vi "1003088 print label from powered unit.vi"(8 "error in (no error)":errorcluster, 10 "Baud":dbl=115200.0, 11 "VISA Refnum in":refnum<visa-resource-name>="COM11") -> (0 "error out":errorcluster)   [LabVIEW 2013]
panel:
  in  "Check label IMEI to unit?":bool
  out "IP":string
  out "Print Label OK?":bool=TRUE
  in  "Serial Number":u32
  in  "Printer name":string="\\\\SkywireTestPC1\\ZDesigner ZT230-300dpi ZPL (Copy 1)"
  out "ZPL final":string
  in  "ZPL template":string="\u0010CT~~CD,~CC^~CT~\n^XA~TA000~JSN^LT0^MNW^MTT^PON^PMN^LH0,0^JMA^PR4,4~SD21^JUS^LRN^CI0^XZ\n^FX Start of label zpl^FS\n^XA\n^MMT\n^PW300\n^LL0300\n^LS0\n^FO30,20^GFA,01536,01536,00024,:Z64:\neJzt0s1Kw0AQAOC0gU3B0iB4EAlppQcvHlKE0kNhX0Uo6EsImVLwB8W+QLBvYtUFexH6AoJKhVwjuaSwdN100tDALiL04ME57OFjdnZ3Zg1jU2FB5Krc/kioyutxQkHpXO1zjXONL85+8AouZuaiS8Ere0s3oSsf5KAH0sm676G/UOgQI/OK9J3cD3NPG7OL/kmhTbYDtxJZA3BOJxd47ltE4YC0xv4WrzNwRDjE/KnsT5O0GKtVvV7qIyP3/fNWv39DjpvgfIX36BPZB+8Z/QicKEzQ2YJC40T6Zbngj2Llph+nztEfUm9jvlnwMXgu1l/6HfqTL6BRk35LvKYIonCYnUszv3Y6PfFadCL9KrGZCN5nVuYjsZpXaX1ebJp7YY4s1PhM47HG5xrnOvd/4/aAK/+/ZfKqyg2TK1nvQiQaV+6QvtiElzT1Dc19/uMPxjcSRcXX:E7E0\n\n^FO190,20^GFA,00256,00256,00008,:Z64:\neJxjYCAZMEFp/g8Q2v4PhK7gg9AJ7BD6/OMGEMV4/iOE7iuE0gUHwHT/Ayh9AEL3QfkwdecswTTDAeYGFHNh9sj/QXUHWQAAi6QYnQ==:D803\n\n^FT75,92^A0N,29,29^FH\\^FDSKYWIRE^FS\n^FO175,60^GFA,00256,00256,00008,:Z64:\neJxjYCAZMEFp/g8Q2v4PhK7gg9AJ7BD6/OMGEMV4/iOE7iuE0gUHwHT/Ayh9AEL3QfkwdecswTTDAeYGFHNh9sj/QXUHWQAAi6QYnQ==:D803\n\n^FT0,115^A@N,20,20,ari001^FH\\^FDP/N: NL-SW-LTE-TC1WWG^FS\n^FT0,139^A@N,23,23,ari001^FH\\^FDIMEI: ImeiImeiImeiIme^FS\n^FT0,163^A@N,19,19,ari001^FH\\^FDICCID:EsimEsimEsimEsimEsim^FS\n^FT0,187^A@N,19,19,ari001^FH\\^FDBTW BTWSNWWYY^FS\n^FT0,211^A@N,24,24,ari001^FH\\^FD1003088 REV A^FS\n^BY56,56^FT203,275^BXN,3,200,0,0,1,~\n^FH\\^FDImeiImeiImeiIme,BTW BTWSNWWYY,EsimEsimEsimEsimEsim^FS\n^PQ1,0,1,Y^XZ"
  out "imei":string
  out "eSim ICCID":string
  # "printer1=\\\\\\\\SkywireTestPC1\\ZDesigner ZT230-300dpi ZPL (Copy 1)\nprinter2=\\\\\\\\PucTestPC2\\ZDesigner ZT230-300dpi ZPL\nprinter3=\\\\\\\\NIMBELNKTESTPC3\\ZDesigner GX430t\nprinter4=\\\\\\\\dt-hkn77p2\\ZDesigner ZT230-200dpi ZPL\nprinter5=\\\\\\\\nimbelink-08\\ZDesigner ZT230-300dpi ZPL\nprinter6=\\\\\\\\LT-85LKFW2\\\\"
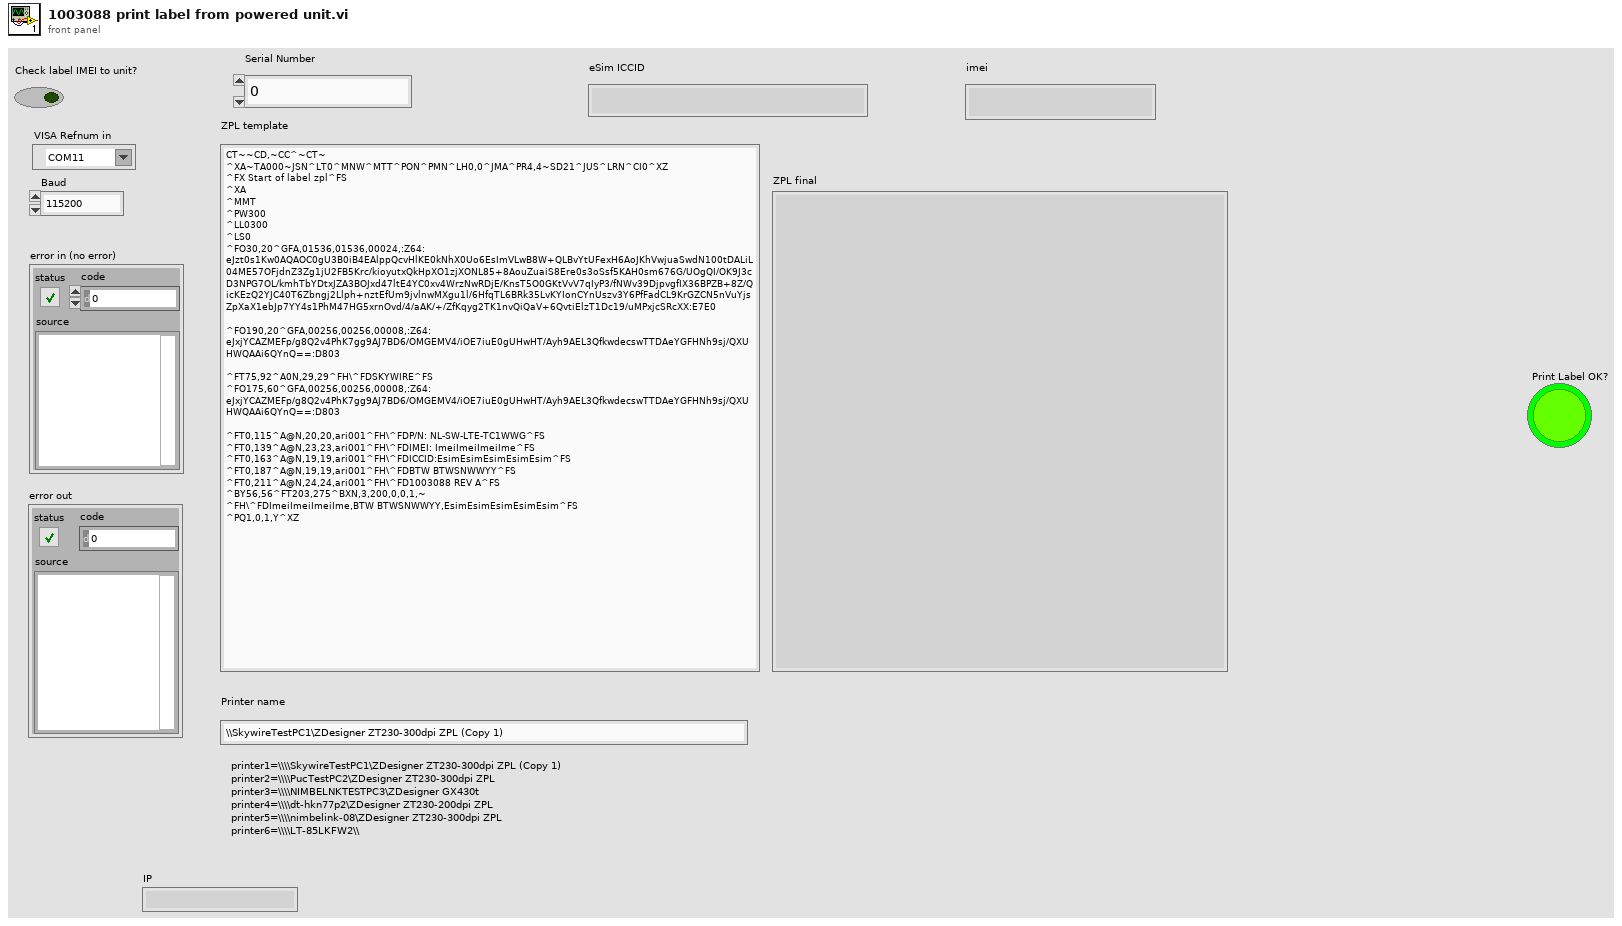
[diagram p1: front panel]
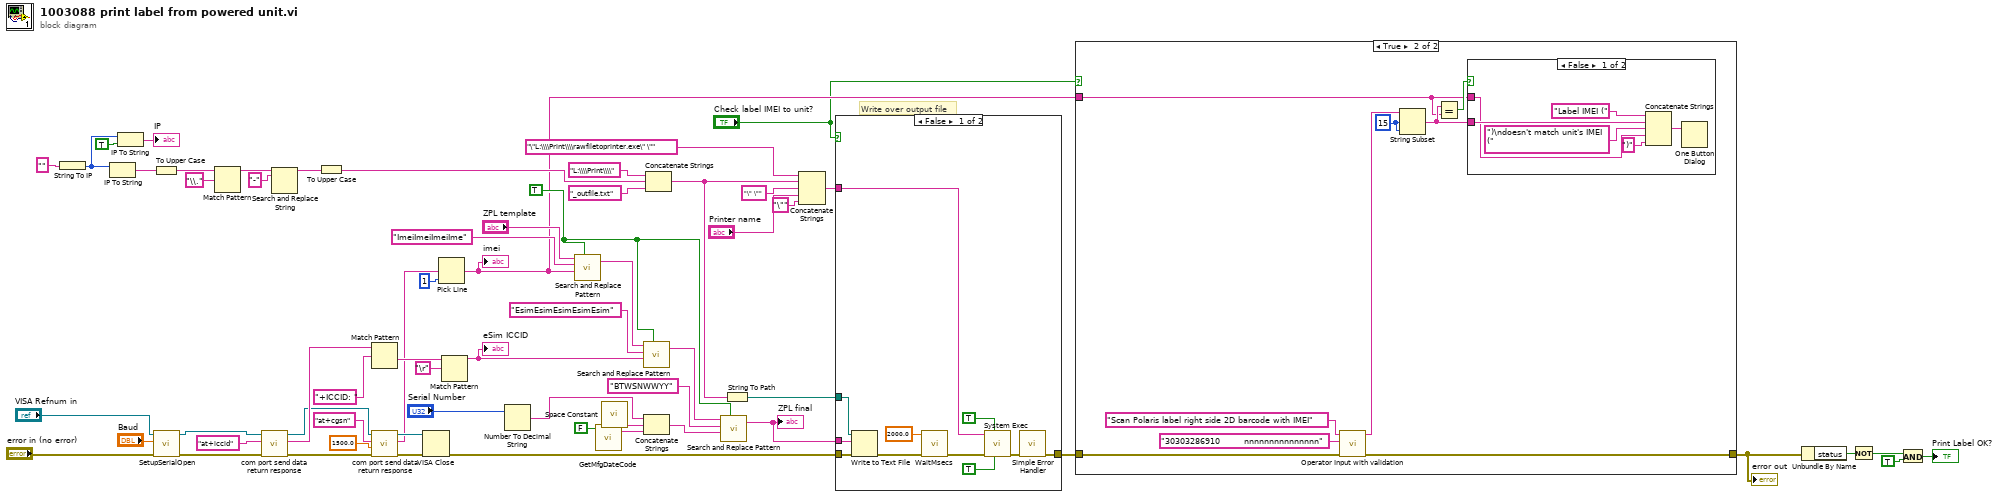
[diagram p0: block diagram]
diagram:
  w44 = TRUE ("replace all? (F)")
  # "Write over output file"
  n1 = String To IP(1:"" ("name")) -> (0:w28:u32)
  n2 = IP To String(2:w28) -> (0:w22:string)  [unwired: 1 in]
  n3 = IP To String(1:TRUE ("dot notation? (F)"), 2:w28) -> (0:→"IP":string)
  n4 = To Upper Case(1:w22) -> (0:w21:string)
  n5 = call "SetupSerialOpen.vi"("error in (no error)"="error in (no error)", "Baud"="Baud", "VISA Refnum in"="VISA Refnum in") -> ("error out"=w59:errorcluster, "VISA session"=w10:refnum<visa-resource-name>)  [unwired: 7 in]
  n6 = Match Pattern(string=w21, regular expression="\\.") -> (before substring=w25:string)  [unwired: 1 in, 3 out]
  n7 = call "com port send data return response.vi"("error in (no error)"=w59, "Send data"="at+iccid", "VISA resource name"=w10) -> ("error out"=w53:errorcluster, "response"=w55:string, "VISA resource name out"=w52:refnum<visa-resource-name>)  [unwired: 5 in, 1 out]
  n8 = Search and Replace String(input string=w25, search string="-") -> (result string=w23:string)  [unwired: 6 in, 3 out]
  n9 = To Upper Case(1:w23) -> (0:w20:string)
  n10 = Match Pattern(string=w55, regular expression="+ICCID: ") -> (after substring=w46:string)  [unwired: 1 in, 3 out]
  n11 = call "com port send data return response.vi"("error in (no error)"=w53, "Wait Msecs for response"=1500.0, "Send data"="at+cgsn", "VISA resource name"=w52) -> ("error out"=w41:errorcluster, "response"=w14:string, "VISA resource name out"=w51:refnum<visa-resource-name>)  [unwired: 4 in, 1 out]
  n12 = VISA Close(VISA resource name=w51, error in (no error)=w41) -> (error out=w17:errorcluster)
  n13 = Pick Line(multi-line string=w14, line index=1) -> (output string=w9:string)  [unwired: 1 in]
  "imei" <- w9
  n14 = Match Pattern(string=w46, regular expression="\r") -> (before substring=w11:string)  [unwired: 1 in, 3 out]
  "eSim ICCID" <- w11
  n15 = Number To Decimal String(number="Serial Number") -> (decimal integer string=w5:string)  [unwired: 1 in]
  n16 = call <vilib>:"Search and Replace Pattern.vi"("string"="ZPL template", "regular expression (\"\")"="ImeiImeiImeiIme" ("string"), "replace string (\"\")"=w9, "replace all? (F)"=w44) -> ("result string"=w48:string)  [unwired: 1 in, 1 out]
  n17 = call "GetMfgDateCode.vi"("quit? (T)"=FALSE) -> ("WeekYearCode"=w2:string)  [unwired: 2 in, 1 out]
  n18 = call <vilib>:"Space Constant.vi"() -> ("String"=w3:string)
  n19 = call <vilib>:"Search and Replace Pattern.vi"("string"=w48, "regular expression (\"\")"="EsimEsimEsimEsimEsim" ("regular expression (\"\")"), "replace string (\"\")"=w11, "replace all? (F)"=w44) -> ("result string"=w45:string)  [unwired: 1 in, 1 out]
  n20 = Concatenate Strings(w5, w3, w2) -> (w4:string)
  n21 = Concatenate Strings("L:\\\\Print\\\\" ("string"), w20, "_outfile.txt" ("string")) -> (w31:string)
  n22 = call <vilib>:"Search and Replace Pattern.vi"("string"=w45, "regular expression (\"\")"="BTWSNWWYY" ("regular expression (\"\")"), "replace string (\"\")"=w4, "replace all? (F)"=w44) -> ("result string"=w16:string)  [unwired: 1 in, 1 out]
  "ZPL final" <- w16
  n23 = String To Path(string=w31) -> (path=w19:path)
  n24 = Concatenate Strings("\"L:\\\\Print\\\\rawfiletoprinter.exe\" \"" ("string"), w31, "\" \"" ("string"), "Printer name", "\"" ("string")) -> (w18:string)
  n25 = case shown="False" "Check label IMEI to unit?" {
    tunnel: w19 -> [w68 _]
    tunnel: w18 -> [w66 _]
    tunnel: w17 -> [w65 w74]
    tunnel: w16 -> [w64 _]
    tunnel: [w63 w74] -> w7
    frame False {
      n26 = Write to Text File(file (use dialog)=w68, text=w64, error in=w65) -> (error out=w67:errorcluster)  [unwired: 1 in, 2 out]
      n27 = call "WaitMsecs.vi"("error in (no error)"=w67, "Wait Msecs"=2000.0) -> ("error out"=w70:errorcluster)  [unwired: 9 in]
      n28 = call <vilib>:"System Exec.vi"("run minimized? (F)"=TRUE, "wait until completion? (T)"=TRUE, "error in (no error)"=w70, "command line"=w66) -> ("error out"=w71:errorcluster)  [unwired: 4 in, 3 out]
      n29 = call <vilib>:"Simple Error Handler.vi"("error in (no error)"=w71) -> ("error out"=w63:errorcluster)  [unwired: 4 in, 4 out]
    }
    frame True {
    }
  }
  n30 = case shown="True" "Check label IMEI to unit?" {
    tunnel: w9 -> [_ w76]
    tunnel: w7 -> [w75 w80]
    tunnel: [w75 w79] -> w6
    frame False {
    }
    frame True {
      w82 = 15 ("offset (0)")
      n31 = call "Operator Input with validation.vi"("error in (no error)"=w80, "Validation string"="30303286910        nnnnnnnnnnnnnnn", "Message"="Scan Polaris label right side 2D barcode with IMEI") -> ("error out"=w79:errorcluster, "Response"=w83:string)  [unwired: 6 in, 1 out]
      n32 = String Subset(string=w83, offset (0)=w82, length (rest)=w82) -> (substring=w77:string)
      n33 = Equal?(x=w77, y=w76) -> (x = y?=w78:bool)
      n34 = case shown="False" w78 {
        tunnel: w77 -> [w89 _]
        tunnel: w76 -> [w87 _]
        frame False {
          n35 = Concatenate Strings("Label IMEI (" ("string"), w89, ")\ndoesn't match unit's IMEI (" ("string"), w87, ")" ("string")) -> (w85:string)
          n36 = One Button Dialog(message=w85) -> ()  [unwired: 1 in, 1 out]
        }
        frame True {
        }
      }
    }
  }
  "error out" <- w6
  n37 = Unbundle By Name(w6) -> ("status"=w38:bool)
  n38 = Not(x=w38) -> (.not. x?=w37:bool)
  n39 = And(x=w37, y=TRUE) -> (x .and. y?=→"Print Label OK?":bool)
